vi "BMark_Create Tree.vi"(6 "Search String":string, 8 "error in (no error)":errorcluster, 9 "GroupByVI":bool, 10 "TreeRef":refnum<vi>, 11 "Bookmark info":T1[](array[typedef])) -> (0 "error out":errorcluster)   [LabVIEW 2013]
uses:
  controls/BMark_Bookmark Data.ctl
  controls/BMark_VI_Identifier.ctl
  <vilib>/addons/analyzer/_analyzerctrls.llb/VIAnCtl Analysis App Info.ctl
  globals/BMark_User Visible Strings.vi
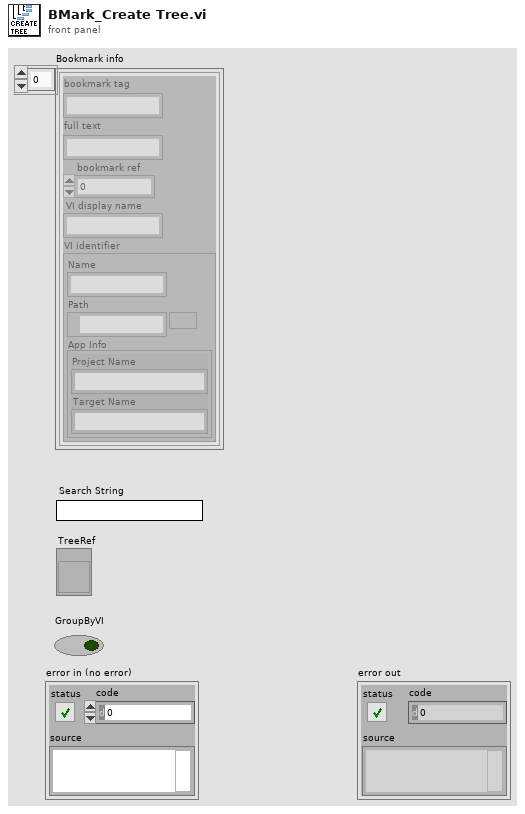
[diagram p1: front panel]
types:
  T1 = typedef "BMark_Bookmark Data.ctl" = cluster{"bookmark tag":string, "full text":string, "bookmark ref":i32, "VI display name":string, "VI identifier":T2}
  T2 = typedef "BMark_VI_Identifier.ctl" = cluster{"Name":string, "Path":path, "App Info":T3}
  T3 = typedef "VIAnCtl Analysis App Info.ctl" = cluster{"Project Name":string, "Target Name":string}
  T4 = enum8{"Enabled", "Disabled", "Disabled and Grayed Out"}
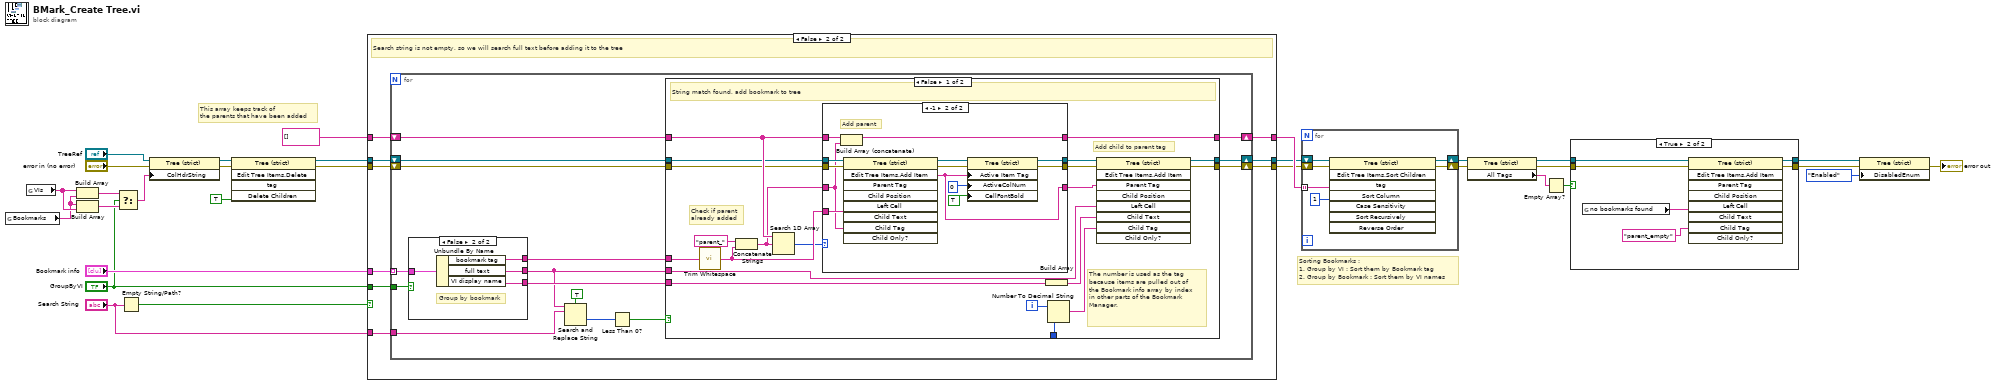
[diagram p0: block diagram]
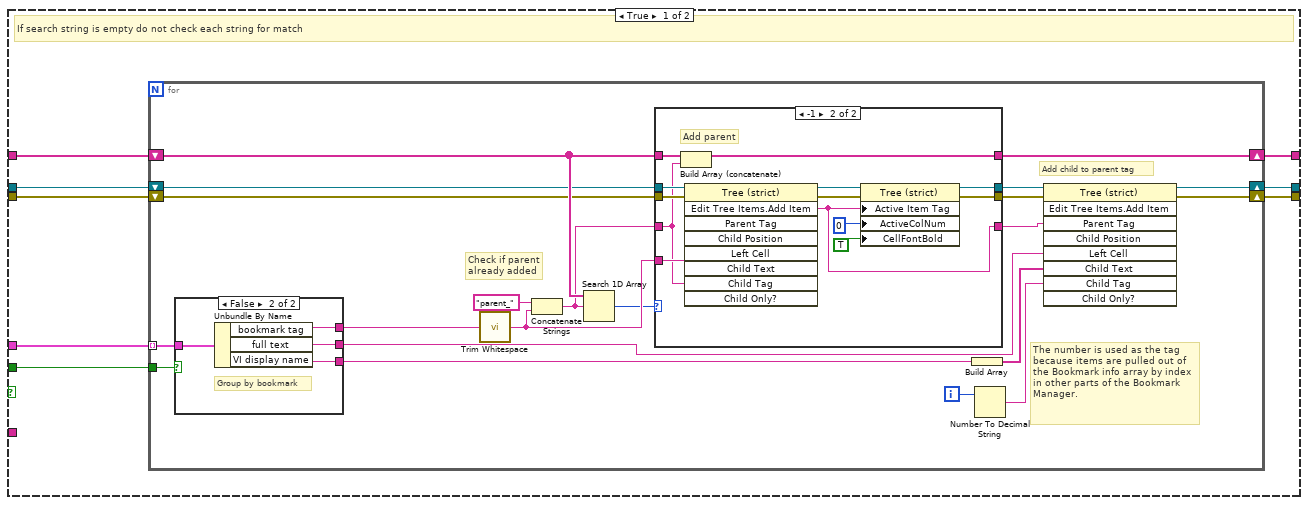
[diagram p2: hidden frame]
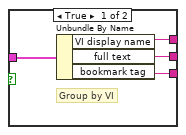
[diagram p4: hidden frame]
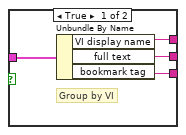
[diagram p7: hidden frame]
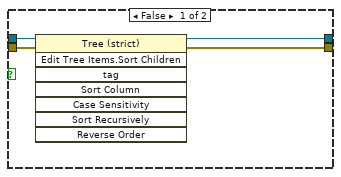
[diagram p8: hidden frame]
diagram:
  # "Sorting Bookmarks :\n1. Group by VI : Sort them by Bookmark tag\n2. Group by Bookmark : Sort them by VI names"
  # "This array keeps track of \nthe parents that have been added"
  n1 = global read "BMark_User Visible Strings.vi" "Bookmarks"() -> (w8:string)
  n2 = global read "BMark_User Visible Strings.vi" "VIs"() -> (w9:string)
  n3 = Build Array(w9, w8) -> (w21:string[])
  n4 = Build Array(w8, w9) -> (w20:string[])
  n5 = Select(t=w21, s="GroupByVI", f=w20) -> (s? t:f=w19:string[])
  n6 = Empty String/Path?(string/path="Search String") -> (empty?=w2:bool)
  n7 = property class="Tree (strict)"(reference="TreeRef", error in="error in (no error)", "ColHdrString"=w19) -> (reference out=w14:refnum<vi>, error out=w15:errorcluster)
  n8 = invoke class="Tree (strict)" method="Edit Tree Items.Delete"(reference=w14, error in=w15, "Delete Children"=TRUE ("Delete Children?")) -> (reference out=w28:refnum<vi>, error out=w29:errorcluster)  [unwired: 2 in, 3 out]
  n9 = case shown="False" w2 {
    tunnel: w29 -> [w38 w93]
    tunnel: w28 -> [w37 w92]
    tunnel: "Bookmark info" -> [w36 w91]
    tunnel: string[] [] -> [w35 w90]
    tunnel: [w34 w89] -> w25
    tunnel: [w33 w88] -> w24
    tunnel: "GroupByVI" -> [w32 w87]
    tunnel: [w31 w86] -> w3
    tunnel: "Search String" -> [_ w85]
    frame True {
      # "If search string is empty do not check each string for match"
      n10 = for {
        tunnel: w36 -> [w59] mode=indexing
        shift-right: [w57] -> w34
        shift-left: w35 -> [w58]
        shift-right: [w54] -> w33
        shift-left: w37 -> [w56]
        tunnel: w32 -> [w51]
        shift-right: [w49] -> w31
        shift-left: w38 -> [w53]
        i -> [w48]
        # "The number is used as the tag because items are pulled out of the Bookmark info array by index in other parts of the Bookmark Manager."
        # "Check if parent\nalready added"
        # "Add child to parent tag"
        n11 = case shown="False" w51 {
          tunnel: w59 -> [w80 w84]
          tunnel: [w79 w83] -> w55
          tunnel: [w78 w82] -> w50
          tunnel: [w77 w81] -> w52
          frame True {
            # "Group by VI"
            n12 = Unbundle By Name(w80) -> ("VI display name"=w78:string, "full text"=w79:string, "bookmark tag"=w77:string)
          }
          frame False {
            # "Group by bookmark"
            n13 = Unbundle By Name(w84) -> ("bookmark tag"=w82:string, "full text"=w83:string, "VI display name"=w81:string)
          }
        }
        n14 = call <vilib>:"Trim Whitespace.vi"("string"=w50) -> ("trimmed string"=w41:string)  [unwired: 1 in]
        n15 = Concatenate Strings("parent_", w41) -> (w43:string)
        n16 = Search 1D Array(1D array=w58, element=w43) -> (index of element=w40:i32)  [unwired: 1 in]
        n17 = case shown="-1" w40 {
          tunnel: w58 -> [w63 w76]
          tunnel: w43 -> [w60 w69]
          tunnel: [w63 w75] -> w57
          tunnel: w53 -> [w61 w73]
          tunnel: [w61 w66] -> w42
          tunnel: w56 -> [w62 w74]
          tunnel: [w62 w65] -> w47
          tunnel: [w60 w64] -> w45
          tunnel: w41 -> [_ w72]
          frame Default {
            # "Tag previously added"
          }
          frame -1 {
            # "Add parent"
            n18 = Build Array (concatenate)(w76, w69) -> (w75:string[])
            n19 = invoke class="Tree (strict)" method="Edit Tree Items.Add Item"(reference=w74, error in=w73, "Left Cell"=w72, "Child Tag"=w69) -> (reference out=w71:refnum<vi>, error out=w70:errorcluster, "Edit Tree Items:Add Item"=w64:string)  [unwired: 5 in, 6 out]
            n20 = property class="Tree (strict)"(reference=w71, error in=w70, "Active Item Tag"=w64, "ActiveColNum"=0 ("Active Cell:Active Column Number"), "CellFontBold"=TRUE ("Active Cell:Cell Font:Bold")) -> (reference out=w65:refnum<vi>, error out=w66:errorcluster)
          }
        }
        n21 = Build Array(w52) -> (w46:string[])
        n22 = Number To Decimal String(number=w48) -> (decimal integer string=w39:string)  [unwired: 1 in]
        n23 = invoke class="Tree (strict)" method="Edit Tree Items.Add Item"(reference=w47, error in=w42, "Parent Tag"=w45, "Left Cell"=w55, "Child Text"=w46, "Child Tag"=w39) -> (reference out=w54:refnum<vi>, error out=w49:errorcluster)  [unwired: 3 in, 7 out]
      }
    }
    frame False {
      # "Search string is not empty, so we will search full text before adding it to the tree"
      n24 = for {
        tunnel: w91 -> [w109] mode=indexing
        shift-right: [w107] -> w89
        shift-left: w90 -> [w108]
        shift-right: [w105] -> w88
        shift-left: w92 -> [w106]
        tunnel: w87 -> [w102]
        shift-right: [w100] -> w86
        shift-left: w93 -> [w104]
        tunnel: w85 -> [w97]
        i -> [w99]
        n25 = case shown="False" w102 {
          tunnel: w109 -> [w152 w156]
          tunnel: [w151 w155] -> w98
          tunnel: [w150 w154] -> w101
          tunnel: [w149 w153] -> w103
          frame True {
            # "Group by VI"
            n26 = Unbundle By Name(w152) -> ("VI display name"=w150:string, "full text"=w151:string, "bookmark tag"=w149:string)
          }
          frame False {
            # "Group by bookmark"
            n27 = Unbundle By Name(w156) -> ("bookmark tag"=w154:string, "full text"=w155:string, "VI display name"=w153:string)
          }
        }
        n28 = Search and Replace String(case sensitive?=TRUE ("ignore case? (F)"), input string=w98, search string=w97) -> (offset past replacement=w96:i32)  [unwired: 5 in, 3 out]
        n29 = Less Than 0?(x=w96) -> (x < 0?=w95:bool)
        n30 = case shown="False" w95 {
          tunnel: w108 -> [w128 w146]
          tunnel: [w127 w146] -> w107
          tunnel: w106 -> [w126 w148]
          tunnel: w98 -> [w125 _]
          tunnel: [w124 w148] -> w105
          tunnel: w104 -> [w123 w147]
          tunnel: w103 -> [w122 _]
          tunnel: w101 -> [w121 _]
          tunnel: [w120 w147] -> w100
          tunnel: w99 -> [w119 _]
          frame False {
            # "The number is used as the tag because items are pulled out of the Bookmark info array by index in other parts of the Bookmark Manager."
            # "Check if parent\nalready added"
            # "Add child to parent tag"
            # "String match found, add bookmark to tree"
            n31 = call <vilib>:"Trim Whitespace.vi"("string"=w121) -> ("trimmed string"=w112:string)  [unwired: 1 in]
            n32 = Concatenate Strings("parent_", w112) -> (w114:string)
            n33 = Search 1D Array(1D array=w128, element=w114) -> (index of element=w111:i32)  [unwired: 1 in]
            n34 = case shown="-1" w111 {
              tunnel: w128 -> [w132 w145]
              tunnel: w114 -> [w129 w138]
              tunnel: [w132 w144] -> w127
              tunnel: w123 -> [w130 w142]
              tunnel: [w130 w135] -> w113
              tunnel: w126 -> [w131 w143]
              tunnel: [w131 w134] -> w118
              tunnel: [w129 w133] -> w116
              tunnel: w112 -> [_ w141]
              frame Default {
                # "Tag previously added"
              }
              frame -1 {
                # "Add parent"
                n35 = Build Array (concatenate)(w145, w138) -> (w144:string[])
                n36 = invoke class="Tree (strict)" method="Edit Tree Items.Add Item"(reference=w143, error in=w142, "Left Cell"=w141, "Child Tag"=w138) -> (reference out=w140:refnum<vi>, error out=w139:errorcluster, "Edit Tree Items:Add Item"=w133:string)  [unwired: 5 in, 6 out]
                n37 = property class="Tree (strict)"(reference=w140, error in=w139, "Active Item Tag"=w133, "ActiveColNum"=0 ("Active Cell:Active Column Number"), "CellFontBold"=TRUE ("Active Cell:Cell Font:Bold")) -> (reference out=w134:refnum<vi>, error out=w135:errorcluster)
              }
            }
            n38 = Build Array(w122) -> (w117:string[])
            n39 = Number To Decimal String(number=w119) -> (decimal integer string=w110:string)  [unwired: 1 in]
            n40 = invoke class="Tree (strict)" method="Edit Tree Items.Add Item"(reference=w118, error in=w113, "Parent Tag"=w116, "Left Cell"=w125, "Child Text"=w117, "Child Tag"=w110) -> (reference out=w124:refnum<vi>, error out=w120:errorcluster)  [unwired: 3 in, 7 out]
          }
          frame True {
          }
        }
      }
    }
  }
  n41 = for {
    tunnel: w25 -> [w161] mode=indexing
    shift-right: [w159] -> w13
    shift-left: w24 -> [w162]
    shift-right: [w160] -> w12
    shift-left: w3 -> [w158]
    n42 = invoke class="Tree (strict)" method="Edit Tree Items.Sort Children"(reference=w162, error in=w158, "tag"=w161, "Sort Column"=1) -> (reference out=w159:refnum<vi>, error out=w160:errorcluster)  [unwired: 4 in, 6 out]
  }
  n43 = property class="Tree (strict)"(reference=w13, error in=w12) -> (reference out=w23:refnum<vi>, error out=w22:errorcluster, "All Tags"=w11:string[])
  n44 = Empty Array?(array=w11) -> (empty?=w10:bool)
  n45 = case shown="True" w10 {
    tunnel: w23 -> [w166 w172]
    tunnel: w22 -> [w165 w171]
    tunnel: [w164 w170] -> w6
    tunnel: [w163 w167] -> w7
    frame False {
      n46 = invoke class="Tree (strict)" method="Edit Tree Items.Sort Children"(reference=w166, error in=w165) -> (reference out=w163:refnum<vi>, error out=w164:errorcluster)  [unwired: 6 in, 6 out]
    }
    frame True {
      n47 = global read "BMark_User Visible Strings.vi" "no bookmarks found"() -> (w168:string)
      n48 = invoke class="Tree (strict)" method="Edit Tree Items.Add Item"(reference=w172, error in=w171, "Left Cell"=w168, "Child Tag"="parent_empty") -> (reference out=w167:refnum<vi>, error out=w170:errorcluster)  [unwired: 5 in, 7 out]
    }
  }
  n49 = property class="Tree (strict)"(reference=w7, error in=w6, "DisabledEnum"=T4."Enabled" ("Disabled")) -> (error out=→"error out":errorcluster)  [unwired: 1 out]
